vi "FlywheelTicksToVelocity.vi"(1 "ticks/100ms":dbl) -> (0 "flywheel_velocity(RPM)":dbl)   [LabVIEW 2019]
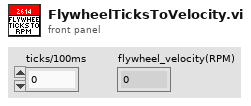
[diagram p1: front panel]
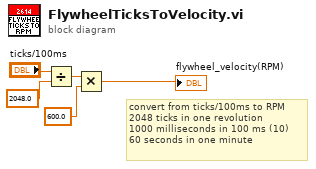
[diagram p0: block diagram]
diagram:
  # "convert from ticks/100ms to RPM\n2048 ticks in one revolution\n1000 milliseconds in 100 ms (10)\n60 seconds in one minute"
  n1 = Divide(x="ticks/100ms", y=2048.0) -> (x/y=w3:dbl)
  n2 = Multiply(x=w3, y=600.0) -> (x*y=→"flywheel_velocity(RPM)":dbl)
